vi "findUserClick.vi"(8 "Error In":errorcluster, 9 "clickLocation":dbl[](array[numeric]), 10 "time_E":dbl[](array[numeric]), 11 "VE_amplitude":dbl[](array[numeric])) -> (0 "Error Out":errorcluster, 2 "amplitudePeaks":dbl[](array[numeric]), 3 "iPeaksLocation":dbl[](array[numeric]) format="%.2f")   [LabVIEW 2012]
doc: "It calculates the i-position and amplitude of peaks that are choosen by the user."
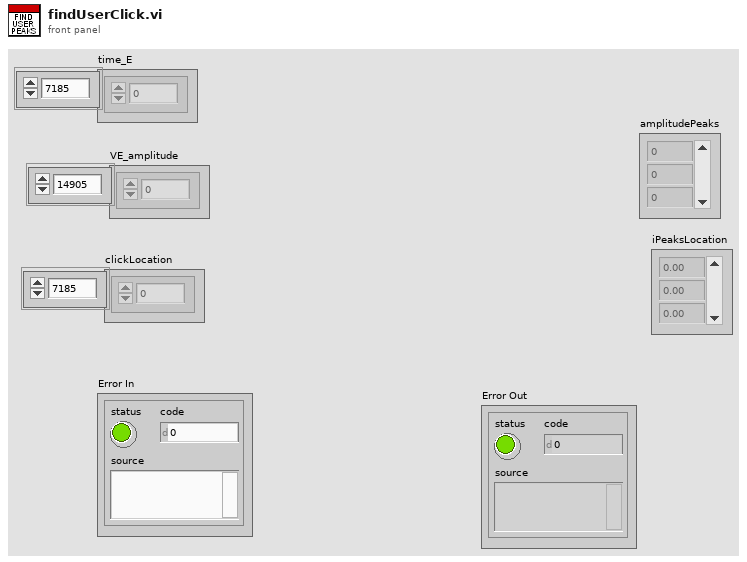
[diagram p1: front panel]
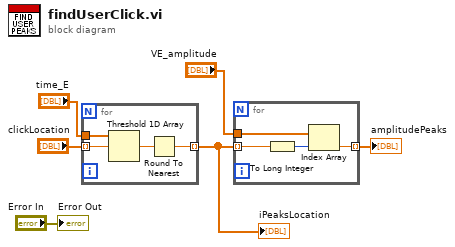
[diagram p0: block diagram]
diagram:
  n1 = for {
    tunnel: "clickLocation" -> [w8] mode=indexing
    tunnel: "time_E" -> [w9]
    tunnel: [w7] -> w1 mode=indexing
    n2 = Threshold 1D Array(2:w8, 3:w9) -> (0:w10:dbl)  [unwired: 1 in]
    n3 = Round To Nearest(number=w10) -> (nearest integer value=w7:dbl)
  }
  "iPeaksLocation" <- w1
  n4 = for {
    tunnel: "VE_amplitude" -> [w14]
    tunnel: w1 -> [w13] mode=indexing
    tunnel: [w11] -> w2 mode=indexing
    n5 = To Long Integer(number=w13) -> (32bit integer=w12:i32)
    n6 = Index Array(array=w14, index=w12) -> (element=w11:dbl)
  }
  "amplitudePeaks" <- w2
  "Error Out" <- "Error In"
